vi "RichToFlatni_measurementlink_discovery_v1_ServiceDescriptor.vi"(5 "OutputClusterType":T1, 11 "InputCluster":T3) -> (3 "OutputCluster":T1)   [LabVIEW 2020, in "Measurement Plugin Discovery Client.lvlib"]
uses:
  Measurement Plugin Discovery Client.lvlib
  ni_measurementlink_discovery_v1_ServiceDescriptor.ctl
  ni_measurementlink_discovery_v1_ServiceDescriptor_AnnotationsEntry.ctl
  ni_measurementlink_discovery_v1_ServiceDescriptor_Flat.ctl
  ni_measurementlink_discovery_v1_ServiceDescriptor_AnnotationsEntry_Flat.ctl
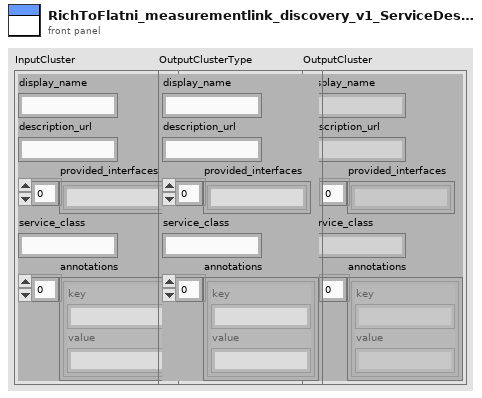
[diagram p1: front panel]
types:
  T1 = typedef "Measurement Plugin Discovery Client.lvlib/ni_measurementlink_discovery_v1_ServiceDescriptor_Flat.ctl" = cluster{"display_name":string, "description_url":string, "provided_interfaces":string[], "service_class":string, "annotations":T2[]}
  T2 = typedef "Measurement Plugin Discovery Client.lvlib/ni_measurementlink_discovery_v1_ServiceDescriptor_AnnotationsEntry_Flat.ctl" = cluster{"key":string, "value":string}
  T3 = typedef "Measurement Plugin Discovery Client.lvlib/ni_measurementlink_discovery_v1_ServiceDescriptor.ctl" = cluster{"display_name":string, "description_url":string, "provided_interfaces":string[], "service_class":string, "annotations":T4[]}
  T4 = typedef "Measurement Plugin Discovery Client.lvlib/ni_measurementlink_discovery_v1_ServiceDescriptor_AnnotationsEntry.ctl" = cluster{"key":string, "value":string}
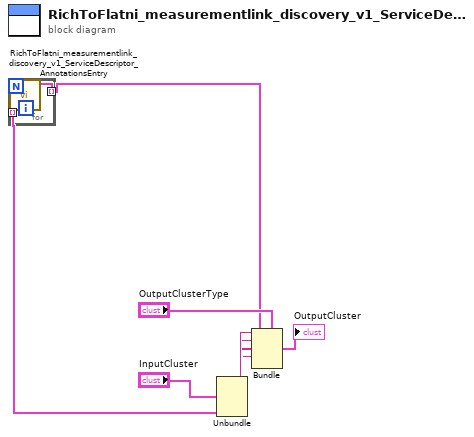
[diagram p0: block diagram]
diagram:
  n1 = Unbundle "Unbundle"("InputCluster") -> ("display_name"=w6:string, "description_url"=w5:string, "provided_interfaces"=w4:string[], "service_class"=w3:string, "annotations"=w2:T4[])
  n2 = for {
    tunnel: w2 -> [w11] mode=indexing
    tunnel: [w10] -> w1 mode=indexing
    n3 = call "RichToFlatni_measurementlink_discovery_v1_ServiceDescriptor_AnnotationsEntry.vi"("InputCluster"=w11) -> ("OutputCluster"=w10:T2)  [unwired: 10 in]
  }
  n4 = Bundle "Bundle"(cluster="OutputClusterType", "display_name"=w6, "description_url"=w5, "provided_interfaces"=w4, "service_class"=w3, "annotations"=w1) -> (→"OutputCluster":T1)
